vi "LaunchTableLogger.vi"(8 "error in (no error)":errorcluster, 9 "Data Cluster (for Headers)":variant, 10 "TableLogger Config":T1={"TableLogger"=enum."SQLite Logger", "DB File Path"=path "DB.db", "DB Backup Interval (Hours)"=24, "Max DB Size (MB)"=100, "Backup Directory"=path "DB/Backup"}, 11 "Parent Actor In (Unwired if root actor)":refnum<class "Actor.lvclass">) -> (0 "error out":errorcluster, 2 "TableLogger Actor's Enqueuer":refnum<class "Message Enqueuer.lvclass">, 3 "Parent Actor Out":refnum<class "Actor.lvclass">, 5 "object out":refnum<class "TableLogger_Actor.lvclass">)   [LabVIEW 2014, in "TableLogger_Actor.lvlib" / "TableLogger_Actor.lvclass"]
uses:
  TableLogger_Actor.lvclass
  <vilib>/ActorFramework/Actor/Actor.lvclass
  TableLoggerConfig.ctl
  TableLoggerTypes.ctl
  <vilib>/ActorFramework/Message Enqueuer/Message Enqueuer.lvclass
  TableLogger_CSV_Actor/TableLogger_CSV_Actor/TableLogger_CSV_Actor.lvclass
  TableLogger_SQLite_Actor/TableLogger_SQLite_Actor/TableLogger_SQLite_Actor.lvclass
  TableLogger_Actor.lvclass/TableLogger_Actor.ctl
  TableLogger_Actor.lvlib
panel:
  # "Connector Pane"
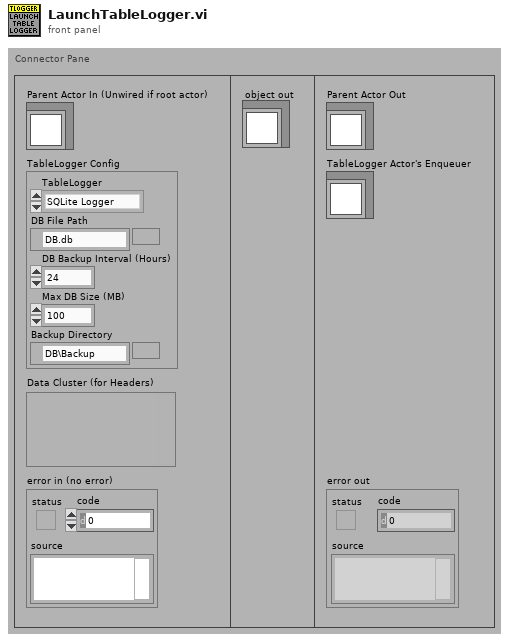
[diagram p1: front panel]
types:
  T1 = typedef "TableLogger_Actor.lvlib/TableLoggerConfig.ctl" = cluster{"TableLogger":T2, "DB File Path":path, "DB Backup Interval (Hours)":i32, "Max DB Size (MB)":i32, "Backup Directory":path}
  T2 = typedef "TableLogger_Actor.lvlib/TableLoggerTypes.ctl" = enum16{"CSV Logger", "SQLite Logger"}
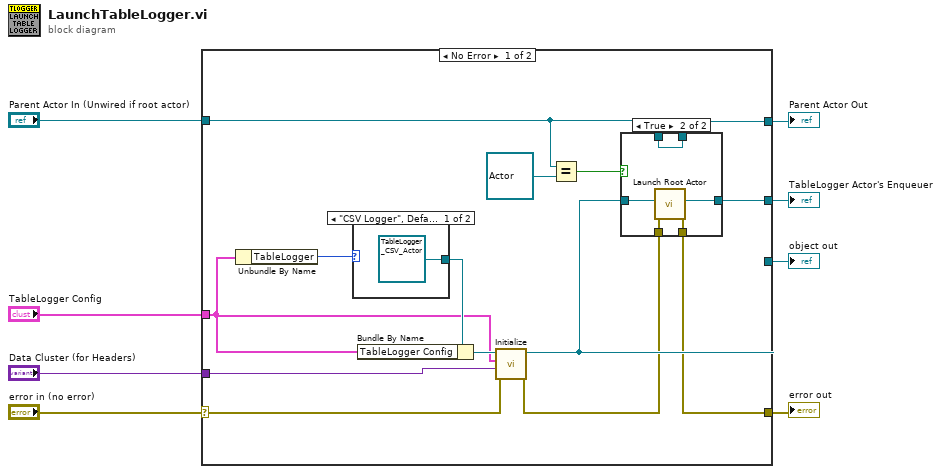
[diagram p0: block diagram]
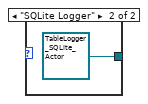
[diagram p2: hidden frame]
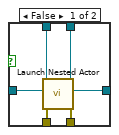
[diagram p3: hidden frame]
diagram:
  n1 = case shown="No Error" "error in (no error)" {
    selector: "error in (no error)" -> [w16 w37]
    tunnel: [w10 w37] -> w7
    tunnel: [w12 _] -> w6
    tunnel: "Parent Actor In (Unwired if root actor)" -> [w14 w36]
    tunnel: "TableLogger Config" -> [w17 _]
    tunnel: "Data Cluster (for Headers)" -> [w15 _]
    tunnel: [w13 w36] -> w2
    tunnel: [w9 _] -> w1
    frame No Error {
      n2 = Unbundle By Name(w17) -> ("TableLogger"=w20:T2)
      n3 = case shown="\"CSV Logger\", Default" w20 {
        tunnel: [refnum<class "TableLogger_CSV_Actor.lvclass"> refnum ("TableLogger_CSV_Actor.lvlib:TableLogger_CSV_Actor.lvclass") refnum<class "TableLogger_SQLite_Actor.lvclass"> refnum ("TableLogger_SQLite_Actor.lvlib:TableLogger_SQLite_Actor.lvclass")] -> w19
        frame "CSV Logger", Default {
        }
        frame "SQLite Logger" {
        }
      }
      n4 = Bundle By Name(cluster=w19, "TableLogger Config"=w17) -> (w18:refnum<class "TableLogger_Actor.lvclass">)
      n5 = call-dynamic "Initialize.vi"("error in (no error)"=w16, "Data Cluster (for Headers)"=w15, "TableLogger Config"=w17, "object in"=w18) -> ("error out"=w11:errorcluster, "object out"=w12:refnum<class "TableLogger_Actor.lvclass">)  [unwired: 6 in]
      n6 = Equal?(x=w14, y=refnum<class "Actor.lvclass"> refnum ("Actor Framework:Actor")) -> (x = y?=w21:bool)
      n7 = case shown="True" w21 {
        tunnel: w14 -> [w30 w35]
        tunnel: [w29 w35] -> w13
        tunnel: w12 -> [w26 w34]
        tunnel: w11 -> [w28 w33]
        tunnel: [w27 w32] -> w10
        tunnel: [w25 w31] -> w9
        frame False {
          n8 = call <vilib>:"Launch Nested Actor.vi"("error in (no error)"=w28, "Nested Actor"=w26, "Caller Actor in"=w30) -> ("error out"=w27:errorcluster, "Nested Actor's Enqueuer"=w25:refnum<class "Message Enqueuer.lvclass">, "Caller Actor out"=w29:refnum<class "Actor.lvclass">)  [unwired: 6 in]
        }
        frame True {
          n9 = call <vilib>:"Launch Root Actor.vi"("error in (no error)"=w33, "Actor"=w34) -> ("error out"=w32:errorcluster, "Actor's Enqueuer"=w31:refnum<class "Message Enqueuer.lvclass">)  [unwired: 8 in]
        }
      }
    }
    frame Error {
    }
  }
  "error out" <- w7
  "object out" <- w6
  "Parent Actor Out" <- w2
  "TableLogger Actor's Enqueuer" <- w1
